vi "Create Sub Events.vi"() -> (2 "Sub Events":T1)   [LabVIEW 2020, in "Vecto.lvlib" / "RemoteDataService.lvclass"]
uses:
  RemoteDataService.lvclass
  RemoteDataService.lvclass/RemoteDataService.ctl
  Subscription Info.ctl
  SubscribedDataHandler/SubscribedDataHandler.lvclass
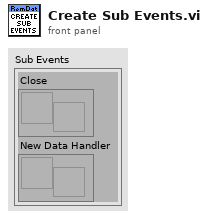
[diagram p1: front panel]
types:
  T1 = typedef "Vecto.lvlib/RemoteDataService.lvclass/Subscription Info.ctl" = cluster{"Close":refnum<user-event>, "New Data Handler":refnum<user-event>}
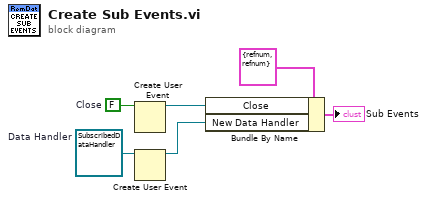
[diagram p0: block diagram]
diagram:
  w3 = refnum<class "SubscribedDataHandler.lvclass"> refnum  # Data Handler
  w6 = FALSE  # Close
  n1 = Create User Event(user event datatype=w6) -> (user event=w4:refnum<user-event>)  [unwired: 1 in, 1 out]
  n2 = Create User Event(user event datatype=w3) -> (user event=w2:refnum<user-event>)  [unwired: 1 in, 1 out]
  n3 = Bundle By Name(cluster=T1 {"Close"=refnum, "New Data Handler"=refnum} ("Subscription Info"), "Close"=w4, "New Data Handler"=w2) -> (→"Sub Events":T1)
